vi "filename_with_timestamp.vi"(11 "filename":string="test") -> (3 "filepath":path)   [LabVIEW 2018]
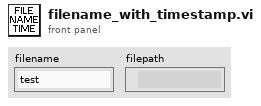
[diagram p1: front panel]
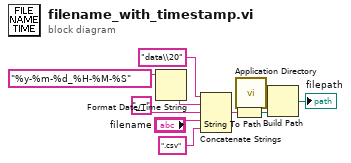
[diagram p0: block diagram]
diagram:
  n1 = Format Date/Time String(time format string (%c)="%y-%m-%d_%H-%M-%S") -> (date/time string=w4:string)  [unwired: 2 in]
  n2 = Concatenate Strings("data\\20" ("string"), w4, "__" ("string"), "filename", ".csv" ("string")) -> (w9:string)
  n3 = String To Path(string=w9) -> (path=w8:path)
  n4 = call <vilib>:"Application Directory.vi"() -> ("Application Directory"=w7:path)
  n5 = Build Path(base path=w7, name or relative path=w8) -> (appended path=→"filepath":path)
